vi "Test_StringToEightByteReal.vi"() -> ()   [LabVIEW 2019]
uses:
  <vilib>/addons/_JKI Toolkits/Caraya/classes/Assert/Assert Almost Equal_Float.vi
  <vilib>/addons/_JKI Toolkits/Caraya/classes/Test/Test.lvclass
  <vilib>/addons/_JKI Toolkits/Caraya/classes/Assert/Assert.lvclass
panel:
  out "error out":errorcluster
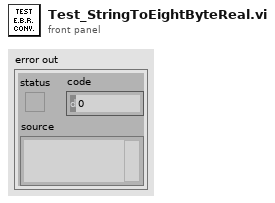
[diagram p1: front panel]
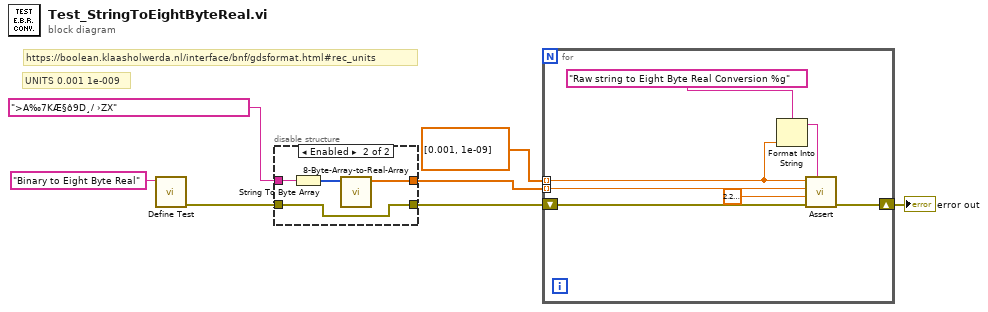
[diagram p0: block diagram]
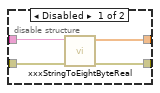
[diagram p2: hidden frame]
diagram:
  # "https://boolean.klaasholwerda.nl/interface/bnf/gdsformat.html#rec_units"
  # "UNITS 0.001 1e-009"
  n1 = call <vilib>:"Define Test.vi"("Label (VI Title)"="Binary to Eight Byte Real") -> ("error out"=w6:errorcluster)  [unwired: 9 in, 1 out]
  n2 = disable-structure shown="Enabled" {
    disable-tunnel: w6 -> [w11 w12]
    disable-tunnel: [w10 w12] -> w5
    disable-tunnel: ">A‰7KÆ§ô9D¸/ ›ZX" -> [w9 w14]
    disable-tunnel: [w8 w13] -> w1
    frame Disabled {
      n3 = call "xxxStringToEightByteReal.vi"("error in (no error)"=w11, "String"=w9) -> ("error out"=w10:errorcluster, "Array"=w8:dbl[])  [unwired: 8 in]
    }
    frame Enabled {
      n4 = String To Byte Array(string=w14) -> (unsigned byte array=w15:u8[])
      n5 = call "8-Byte-Array-to-Real-Array.vi"("Data"=w15) -> ("Array of Values"=w13:dbl[])  [unwired: 10 in]
    }
  }
  n6 = for {
    shift-right: [w21] -> w4
    shift-left: w5 -> [w22]
    tunnel: w1 -> [w20] mode=indexing
    tunnel: dbl[] [0.001, 1e-09] -> [w16] mode=indexing
    n7 = Format Into String(format string="Raw string to Eight Byte Real Conversion %g" ("Label"), w16) -> (resulting string=w19:string)  [unwired: 2 in, 1 out]
    n8 = call-poly <vilib>:"Assert.vi"("Label"=w19, "error in (no error)"=w22, "Tolerance"=2.220446049250313e-16, "Y"=w20, "X"=w16) -> ("error out"=w21:errorcluster)  [unwired: 5 in, 1 out]
  }
  "error out" <- w4
